vi "Handle Type.vi"(8 "error in (no error)":errorcluster, 9 "Type":refnum<class>, 10 "JSON":string, 11 "Flatten To JSON Object in":refnum<class "Flatten To JSON Object.lvclass">) -> (0 "error out":errorcluster, 2 "JSON out":string, 3 "Flatten To JSON Object out":refnum<class "Flatten To JSON Object.lvclass">)   [LabVIEW 2017, in "Flatten To JSON Object.lvclass"]
doc: "Adds type information to the JSON object."
uses:
  Flatten To JSON Object.lvclass
  Flatten To JSON Object.lvclass/Flatten To JSON Object.ctl
  Default Serialization Binder/Default Serialization Binder.lvclass
  C:/Users/de200256/Code/logmanoriginal/jsontext-object-serialization/Serialization Binder/Serialization Binder.lvclass
  <vilib>/JDP Science/JSONtext/Get all Object Items.vi
  <vilib>/JDP Science/JSONtext/Set Multiple Object Items.vi
  Serialization Binder/Serialization Binder.lvclass
  <vilib>/JDP Science/JSONtext/JSONtext.lvlib
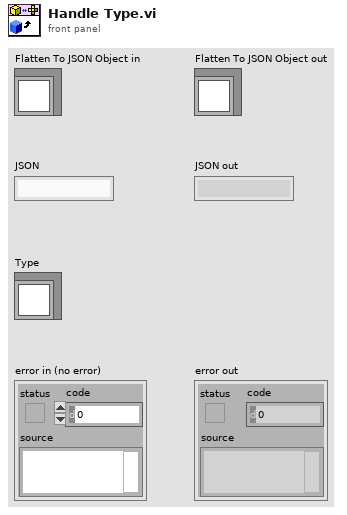
[diagram p1: front panel]
types:
  T1 = typedef "Flatten To JSON Object.lvclass/Type Name Handling.ctl" = enum16{"None", "Inline"}
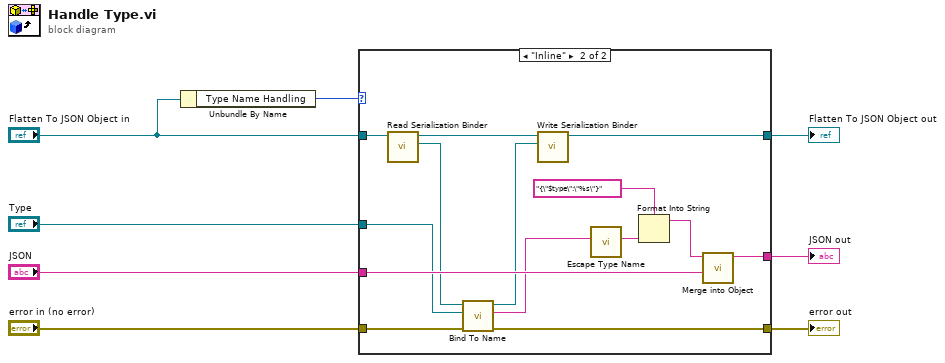
[diagram p0: block diagram]
diagram:
  n1 = Unbundle By Name("Flatten To JSON Object in") -> ("Type Name Handling"=w6:T1)
  n2 = case shown="\"Inline\"" w6 {
    tunnel: [w11 w20] -> w8
    tunnel: "Flatten To JSON Object in" -> [w11 w21]
    tunnel: "Type" -> [_ w19]
    tunnel: "JSON" -> [w10 w22]
    tunnel: [w10 w25] -> w3
    tunnel: "error in (no error)" -> [w9 w15]
    tunnel: [w9 w14] -> w1
    frame Default {
    }
    frame "Inline" {
      n3 = call "Read Serialization Binder.vi"("Flatten To JSON Object in"=w21) -> ("Serialization Binder"=w18:refnum<class "Serialization Binder.lvclass">, "Flatten To JSON Object out"=w16:refnum<class "Flatten To JSON Object.lvclass">)  [unwired: 8 in, 1 out]
      n4 = call-dynamic "Bind To Name.vi"("error in (no error)"=w15, "Type"=w19, "Serialization Binder in"=w18) -> ("error out"=w14:errorcluster, "Type Name"=w12:string, "Serialization Binder out"=w17:refnum<class "Serialization Binder.lvclass">)  [unwired: 6 in]
      n5 = call "Write Serialization Binder.vi"("Serialization Binder"=w17, "Flatten To JSON Object in"=w16) -> ("Flatten To JSON Object out"=w20:refnum<class "Flatten To JSON Object.lvclass">)  [unwired: 8 in, 1 out]
      n6 = call "Escape Type Name.vi"("String"=w12) -> ("String out"=w13:string)  [unwired: 10 in]
      n7 = Format Into String(format string="{\"$type\":\"%s\"}", w13) -> (resulting string=w23:string)  [unwired: 2 in, 1 out]
      n8 = call <vilib>:"Merge into Object.vi"("JSON Object to Merge"=w22, "JSON"=w23) -> ("<JSON>"=w25:string)  [unwired: 7 in, 1 out]
    }
  }
  "error out" <- w1
  "Flatten To JSON Object out" <- w8
  "JSON out" <- w3
